vi "Kyle's Panel.vi"() -> ()   [LabVIEW 2012]
uses:
  Global/GPIB Numbers.vi
panel:
  out "Actual Current":dbl format="%.2f"
  out "Actual Voltage":dbl format="%.2f"
  out "error out":errorcluster
  in  "On?":bool
  in  "Desired Current":dbl format="%.2f"
  in  "Desired Voltage":dbl format="%.2f"
  in  "error in (no error)":errorcluster
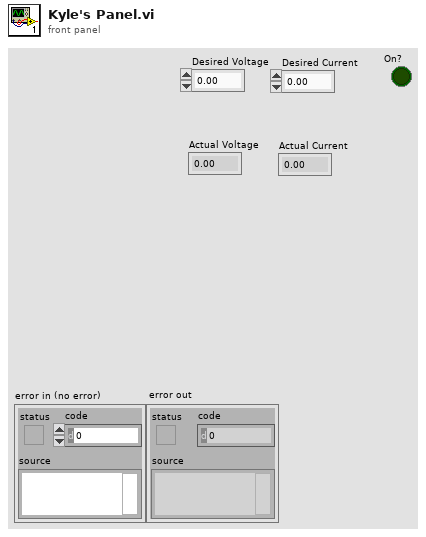
[diagram p1: front panel]
types:
  T1 = cluster{"Name":string, "bus":dbl, "GPIB":dbl, "GPIB as string":string, "byte":i32, "IVI resource name":refnum<k15>, "VISA Resource Name":refnum<visa-resource-name>}
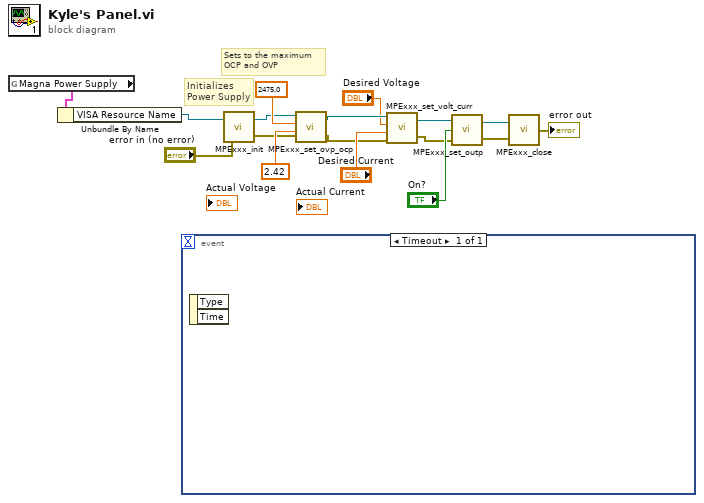
[diagram p0: block diagram]
diagram:
  # "Initializes\nPower Supply"
  # "Sets to the maximum\nOCP and OVP"
  n1 = global read "GPIB Numbers.vi" "Magna Power Supply"() -> (w17:T1)
  n2 = Unbundle By Name(w17) -> ("VISA Resource Name"=w5:refnum<visa-resource-name>)
  n3 = event shown="[0] Timeout" {
    selector: _ -> [_]
    dyn-events: _ -> [_]
    timeout: _ -> [_]
    event Timeout {
      n4 = event-data() -> ()  [unwired: 1 in, 2 out]
    }
  }
  n5 = call "MPExxx_init.vi"("error in (no error)"="error in (no error)", "VISA session"=w5) -> ("error out"=w6:errorcluster, "dup VISA session"=w7:refnum<visa-resource-name>)
  n6 = call "MPExxx_set_ovp_ocp.vi"("error in (no error)"=w6, "Set OCP"=2.42 ("OCP"), "Set OVP"=2475.0 ("OVP"), "VISA session"=w7) -> ("error out"=w12:errorcluster, "dup VISA session"=w13:refnum<visa-resource-name>)
  n7 = call "MPExxx_set_volt_curr.vi"("error in (no error)"=w12, "Set Current"="Desired Current", "Set Voltage"="Desired Voltage", "VISA session"=w13) -> ("error out"=w10:errorcluster, "dup VISA session"=w9:refnum<visa-resource-name>)
  n8 = call "MPExxx_set_outp.vi"("error in (no error)"=w10, "Output Control"="On?", "VISA session"=w9) -> ("error out"=w4:errorcluster, "dup VISA session"=w3:refnum<visa-resource-name>)
  n9 = call "MPExxx_close.vi"("error in (no error)"=w4, "VISA session"=w3) -> ("error out"=→"error out":errorcluster)
